vi "CalculateFilePath (SubVI).vi"(8 "Routines":T1[](array[typedef])=[enum."Score Scale"], 9 "Scale":bool, 10 "OurSwitch":bool, 11 "Position":i32) -> (3 "Flie Path":string)   [LabVIEW 2017]
uses:
  AutonomousRoutine.ctl
  34594ade-77e1-4f4c-b133-a603618e62e1.vi
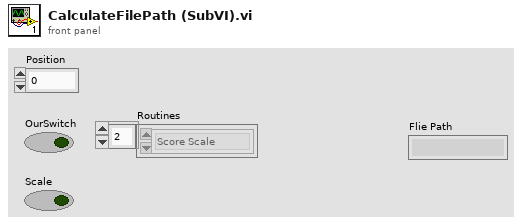
[diagram p1: front panel]
types:
  T1 = typedef "AutonomousRoutine.ctl" = enum16{"Score Scale", "Score Switch"}
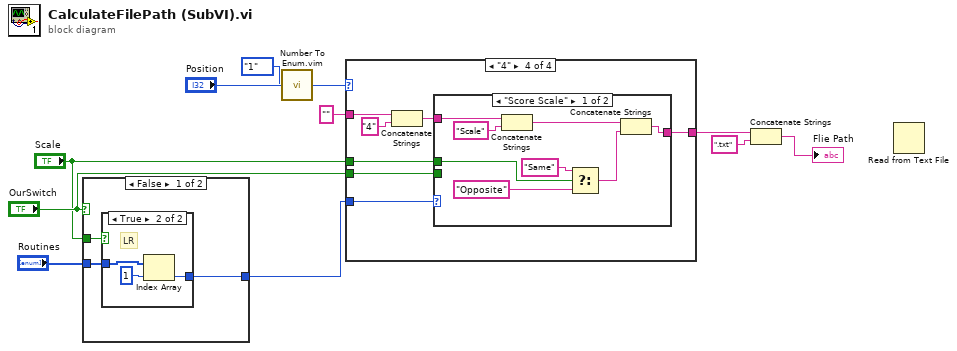
[diagram p0: block diagram]
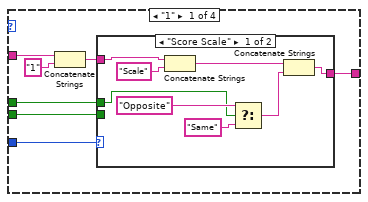
[diagram p2: hidden frame]
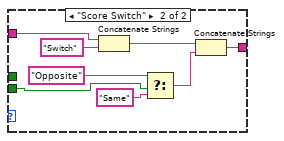
[diagram p3: hidden frame]
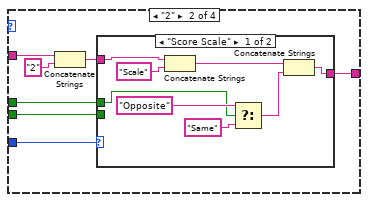
[diagram p4: hidden frame]
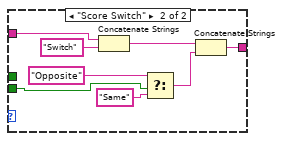
[diagram p5: hidden frame]
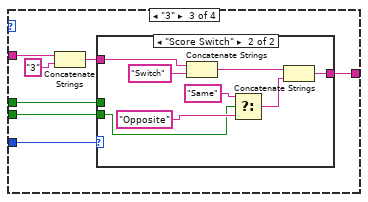
[diagram p6: hidden frame]
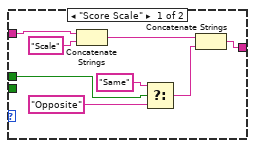
[diagram p7: hidden frame]
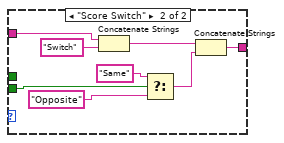
[diagram p8: hidden frame]
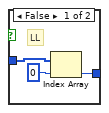
[diagram p9: hidden frame]
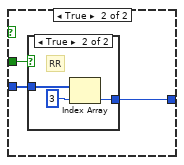
[diagram p10: hidden frame]
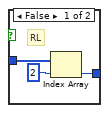
[diagram p11: hidden frame]
diagram:
  n1 = case shown="False" "OurSwitch" {
    tunnel: "Scale" -> [w14 w23]
    tunnel: "Routines" -> [w13 w22]
    tunnel: [w12 w21] -> w3
    frame False {
      n2 = case shown="True" w14 {
        tunnel: w13 -> [w17 w20]
        tunnel: [w15 w18] -> w12
        frame False {
          # "LL"
          n3 = Index Array(array=w17, index=0) -> (element=w15:T1)
        }
        frame True {
          # "LR"
          n4 = Index Array(array=w20, index=1) -> (element=w18:T1)
        }
      }
    }
    frame True {
      n5 = case shown="True" w23 {
        tunnel: w22 -> [w26 w29]
        tunnel: [w24 w27] -> w21
        frame False {
          # "RL"
          n6 = Index Array(array=w26, index=2) -> (element=w24:T1)
        }
        frame True {
          # "RR"
          n7 = Index Array(array=w29, index=3) -> (element=w27:T1)
        }
      }
    }
  }
  n8 = call "Number To Enum.vim"("number"="Position", "enum type"=enum16{"1", "2", "3", "4"}."1" ("Position")) -> ("number as enum"=w5:enum16{"1", "2", "3", "4"})
  n9 = case shown="\"4\"" w5 {
    tunnel: w3 -> [w36 w59 w82 w105]
    tunnel: "OurSwitch" -> [w35 w58 w81 w104]
    tunnel: "Scale" -> [w34 w57 w80 w103]
    tunnel: "" -> [w33 w56 w79 w102]
    tunnel: [w30 w53 w76 w99] -> w11
    frame "1" {
      n10 = Concatenate Strings(w33, "1") -> (w31:string)
      n11 = case shown="\"Score Scale\"" w36 {
        tunnel: w35 -> [_ w49]
        tunnel: w34 -> [w41 _]
        tunnel: w31 -> [w40 w48]
        tunnel: [w38 w46] -> w30
        frame "Score Scale" {
          n12 = Concatenate Strings(w40, "Scale" ("string")) -> (w37:string)
          n13 = Select(t="Opposite", s=w41, f="Same") -> (s? t:f=w42:string)
          n14 = Concatenate Strings(w37, w42) -> (w38:string)
        }
        frame "Score Switch" {
          n15 = Concatenate Strings(w48, "Switch" ("string")) -> (w45:string)
          n16 = Select(t="Opposite", s=w49, f="Same") -> (s? t:f=w50:string)
          n17 = Concatenate Strings(w45, w50) -> (w46:string)
        }
      }
    }
    frame "2" {
      n18 = Concatenate Strings(w56, "2") -> (w54:string)
      n19 = case shown="\"Score Scale\"" w59 {
        tunnel: w58 -> [_ w72]
        tunnel: w57 -> [w65 _]
        tunnel: w54 -> [w62 w70]
        tunnel: [w64 w73] -> w53
        frame "Score Scale" {
          n20 = Concatenate Strings(w62, "Scale" ("string")) -> (w63:string)
          n21 = Select(t="Opposite", s=w65, f="Same") -> (s? t:f=w60:string)
          n22 = Concatenate Strings(w63, w60) -> (w64:string)
        }
        frame "Score Switch" {
          n23 = Concatenate Strings(w70, "Switch" ("string")) -> (w71:string)
          n24 = Select(t="Opposite", s=w72, f="Same") -> (s? t:f=w68:string)
          n25 = Concatenate Strings(w71, w68) -> (w73:string)
        }
      }
    }
    frame "3" {
      n26 = Concatenate Strings(w79, "3") -> (w77:string)
      n27 = case shown="\"Score Switch\"" w82 {
        tunnel: w81 -> [_ w95]
        tunnel: w80 -> [w88 _]
        tunnel: w77 -> [w85 w93]
        tunnel: [w87 w96] -> w76
        frame "Score Scale" {
          n28 = Concatenate Strings(w85, "Scale" ("string")) -> (w86:string)
          n29 = Select(t="Same", s=w88, f="Opposite") -> (s? t:f=w83:string)
          n30 = Concatenate Strings(w86, w83) -> (w87:string)
        }
        frame "Score Switch" {
          n31 = Concatenate Strings(w93, "Switch" ("string")) -> (w94:string)
          n32 = Select(t="Same", s=w95, f="Opposite") -> (s? t:f=w91:string)
          n33 = Concatenate Strings(w94, w91) -> (w96:string)
        }
      }
    }
    frame "4" {
      n34 = Concatenate Strings(w102, "4") -> (w100:string)
      n35 = case shown="\"Score Scale\"" w105 {
        tunnel: w104 -> [_ w118]
        tunnel: w103 -> [w111 _]
        tunnel: w100 -> [w108 w116]
        tunnel: [w110 w119] -> w99
        frame "Score Scale" {
          n36 = Concatenate Strings(w108, "Scale" ("string")) -> (w109:string)
          n37 = Select(t="Same", s=w111, f="Opposite") -> (s? t:f=w106:string)
          n38 = Concatenate Strings(w109, w106) -> (w110:string)
        }
        frame "Score Switch" {
          n39 = Concatenate Strings(w116, "Switch" ("string")) -> (w117:string)
          n40 = Select(t="Same", s=w118, f="Opposite") -> (s? t:f=w114:string)
          n41 = Concatenate Strings(w117, w114) -> (w119:string)
        }
      }
    }
  }
  n42 = Concatenate Strings(w11, ".txt") -> (→"Flie Path":string)
  n43 = Read from Text File() -> ()  [unwired: 4 in, 4 out]
